vi "BW_menu_set (SubVI).vi"(10 "MenuRef":refnum<k9>, 11 "String":string) -> ()   [LabVIEW 2017]
uses:
  st_str Global.vi
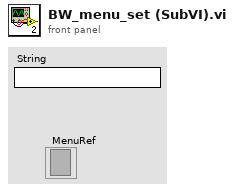
[diagram p1: front panel]
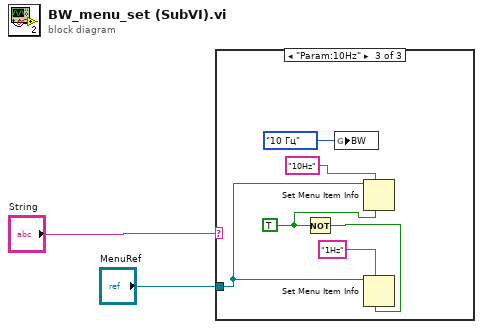
[diagram p0: block diagram]
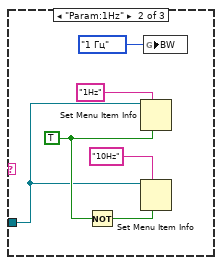
[diagram p3: hidden frame]
diagram:
  n1 = case shown="\"Param:10Hz\"" "String" {
    tunnel: "MenuRef" -> [_ w5 w10]
    frame "False", Default {
    }
    frame "Param:1Hz" {
      w6 = TRUE
      n2 = Not(x=w6) -> (.not. x?=w7:bool)
      n3 = Set Menu Item Info(6:w6, 7:"1Hz" ("item tag"), 11:w5) -> ()  [unwired: 4 in, 2 out]
      n4 = Set Menu Item Info(6:w7, 7:"10Hz" ("item tag"), 11:w5) -> ()  [unwired: 4 in, 2 out]
      n5 = global write "st_str Global.vi" "BW"(enum16{"1 Гц", "10 Гц"}."1 Гц" ("BW")) -> ()
    }
    frame "Param:10Hz" {
      w12 = TRUE ("x")
      n6 = Not(x=w12) -> (.not. x?=w13:bool)
      n7 = global write "st_str Global.vi" "BW"(enum16{"1 Гц", "10 Гц"}."10 Гц" ("BW")) -> ()
      n8 = Set Menu Item Info(6:w12, 7:"10Hz" ("item tag"), 11:w10) -> ()  [unwired: 4 in, 2 out]
      n9 = Set Menu Item Info(6:w13, 7:"1Hz" ("item tag"), 11:w10) -> ()  [unwired: 4 in, 2 out]
    }
  }
